vi "Set Region.vi"(8 "error in (no error)":errorcluster, 10 "Baud Rate":u32=38400, 11 "COM Port":refnum<visa-resource-name>="COM4") -> (0 "error out":errorcluster, 1 "received str":string, 3 "Result":bool)   [LabVIEW 2018]
panel:
  in  "Region":u8=8 format="%x"
  # "SET REGION"
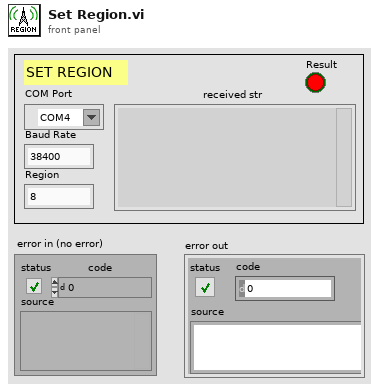
[diagram p1: front panel]
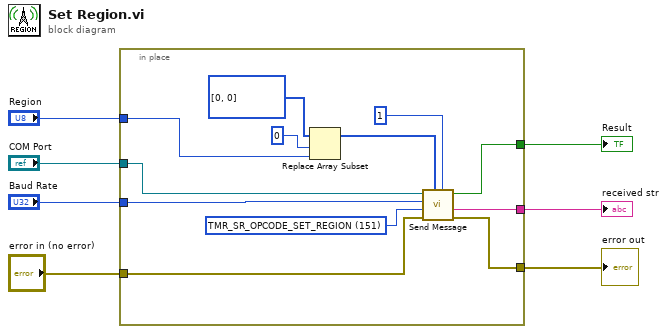
[diagram p0: block diagram]
diagram:
  n1 = in-place {
    in-place-border: "Baud Rate" -> [w19]
    in-place-border: "COM Port" -> [w18]
    in-place-border: "error in (no error)" -> [w16]
    in-place-border: [w15] -> w4
    in-place-border: [w14] -> w3
    in-place-border: [w13] -> w2
    in-place-border: "Region" -> [w8]
    w17 = u16 151 items=["TMR_SR_OPCODE_VERSION"=3, "TMR_SR_OPCODE_SET_BAUD_RATE"=6, "TMR_SR_OPCODE_READ_TAG_ID_SINGLE"=33, "TMR_SR_OPCODE_READ_TAG_ID_MULTIPLE"=34, "TMR_SR_OPCODE_WRITE_TAG_ID"=35, "TMR_SR_OPCODE_WRITE_TAG_DATA"=36, "TMR_SR_OPCODE_KILL_TAG"=38, "TMR_SR_OPCODE_READ_TAG_DATA"=40, "TMR_SR_OPCODE_CLEAR_TAG_ID_BUFFER"=42, "TMR_SR_OPCODE_MULTI_PROTOCOL_TAG_OP"=47, "TMR_SR_OPCODE_GET_READ_TX_POWER"=98, "TMR_SR_OPCODE_GET_WRITE_TX_POWER"=100, "TMR_SR_OPCODE_GET_POWER_MODE"=104, "TMR_SR_OPCODE_GET_READER_OPTIONAL_PARAMS"=106, "TMR_SR_OPCODE_GET_PROTOCOL_PARAM"=107, "TMR_SR_OPCODE_SET_ANTENNA_PORT"=145, "TMR_SR_OPCODE_SET_TAG_PROTOCOL"=147, "TMR_SR_OPCODE_SET_READ_TX_POWER"=146, "TMR_SR_OPCODE_SET_WRITE_TX_POWER"=148, "TMR_SR_OPCODE_SET_REGION"=151, "TMR_SR_OPCODE_SET_READER_OPTIONAL_PARAMS"=154, "TMR_SR_OPCODE_SET_PROTOCOL_PARAM"=155] ("Opcode Constant")
    n2 = Replace Array Subset(array=u8[] [0, 0], new element=w8, index=0) -> (w10:u8[])
    n3 = call "Send Message.vi"("Size"=1, "Data"=w10, "error in (no error)"=w16, "Opcode"=w17, "Baud Rate"=w19, "COM Port"=w18) -> ("error out"=w15:errorcluster, "received str"=w13:string, "Result"=w14:bool)  [unwired: 2 in, 1 out]
  }
  "error out" <- w4
  "Result" <- w3
  "received str" <- w2
